vi "PPWV Partial Pressure of Water Vapor (Pa).vi"(1 "Tceg":dbl[unit], 2 "RH":dbl) -> (0 "PPWV":dbl[unit])   [LabVIEW 2018]
panel:
  out "PPWV\nPartial Pressure of Water\nVapor in Humid-Air(Pa);\nPPWV=(SVP*RH)/100;":dbl[unit](knob)
  out "Temprature Of Input Air\nCentigrade Degree":dbl[unit](slide) scale=0.0..100.0
  out "Humidity of Input Air":dbl(knob) scale=0.0..100.0
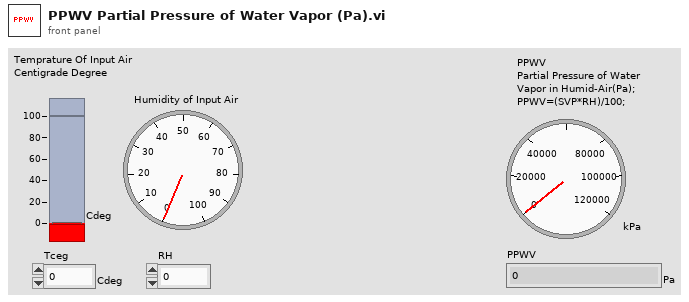
[diagram p1: front panel]
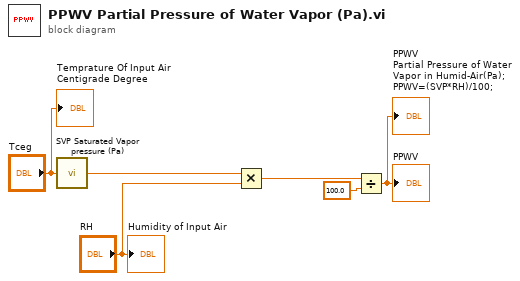
[diagram p0: block diagram]
diagram:
  n1 = call "SVP Saturated Vapor pressure (Pa).vi"("Tceg"="Tceg") -> ("SVP"=w1:dbl[unit])
  n2 = Multiply(x=w1, y="RH") -> (x*y=w5:dbl[unit])
  n3 = Divide(x=w5, y=100.0) -> (x/y=→"PPWV\nPartial Pressure of Water\nVapor in Humid-Air(Pa);\nPPWV=(SVP*RH)/100;" →"PPWV":dbl[unit])
  "Humidity of Input Air" <- "RH"
  "Temprature Of Input Air\nCentigrade Degree" <- "Tceg"
